vi "DOE Parse Temperature and Voltage.vi"(7 "Test Fixture Hardware":T1={"Power "={"Yokogawa"={"WT210"={"Sample Rate (1: 0.25s)"=1, "A Range (12: 20A)"=11, "V Range (6: 600V)"=4, "Power VISA Yokogawa WT210"="WT210"}, "WT500"={"Power VISA Yokogawa WT500"="", "V Range (8: 1000V)"=6, "I Range (7: 40A)"=7, "Update Rate (3: 500ms)"=2}, "WT310_2"={"Sample Rate (1: 0.25s)"=1, "A Range (12: 20A)"=11, "V Range (6: 600V)"=4, "Power VISA Yokogawa WT310_2"="WT310_2"}, "WT310_3"={"Sample Rate (1: 0.25s)"=1, "A Range (12: 20A)"=11, "V Range (6: 600V)"=4, "Power VISA Yokogawa WT310_3"="WT310_3"}}, "Aplus"={"Aplus IP Address"="192.168.1.101", "Remote Port"=502, "Instrument"="APLUS", "Instr Driver Revision"="1.03.0053"}, "Power Limits"={"Crest Factor"={"Upper Limit"=1.49, "Lower Limit"=1.34}, "Harmonic Content"={"Uthd"=2.0}, "Voltage"={"% Error"=2.0}, "Stability"={"<1 Watt "={"Wattage"=1.0, "Slope (mW/H)"=10.0}, ">1 Watt"={"1%Power/Hour"=1.0}}}, "Nominal Voltage"=120, "Time Limit (s)"=10800.0, "Power Variation Limit (%)"=50.0, "Power Supply"={"Chroma 61605"="CHROMA", "Use Chroma?"=FALSE}}, "Weight Scale"={"Com Options"={"IND560Scale VISA"="IND560", "IP Address"="", "Remote Port"=502, "Setra Scale VISA"="SETRA", "GSE 350"="GSE350"}, "Select Scale"=""}, "Flow Rates"={"Laurel Cold IP Address"="", "Laurel Hot IP Address"="", "Hot Water Laurel VISA"="LaurelMeter_Hot", "Cold Water Laurel VISA"="LaurelMeter_Cold", "Remote Port"=0, "Laurel Communication Type"="", "Meters To Collect (Hot Cold)"="", "HOT Laurel Reference"=refnum, "COLD Laurel Reference"=refnum}, "Analog Data"={"Agilent"={"Agilent 34972_1"="34972A_1", "Agilent 34972_2"="34972A_2", "Agilent 34972_3"="34972A_3", "Agilent 34972_4"="34972A_3", "Agilent 34972_5"="34972A_3", "Agilent 34972_6"="34972A_3", "Agilent Gain"=0.0, "TC Type (K,J,T)"="", "Instrument IDN?"="", "TC Channels-List"="", "Analog Channels-List"="", "Agilent Cluster Array"=[], "TC Channels-List 2"="", "Analog Channels-List 2"=""}, "Yokogawa"={"MW100"="MW100", "Intellifaucet"=FALSE}, "Select Analog"="", "TC Coefficients"={"TC Coefficients 1"=[], "TC Coefficients 2"=[], "TC Coefficients 3"=[], "TC Coefficients 4"=[], "TC Coefficients 5"=[], "TC Coefficients 6"=[], "TC Coefficients 7"=[]}, "NI Tasks (Dryer DOE)"=["TC Temps-Module 1", "TC Temps-Module 2", "TC Temps-Module 3", "TC Temps-Module 4", "TC Temps-Module 5", "Gas and Temp-Module 6", "AC_DC Events-Module 7"], "Laurel Analog"={"Laurel IP (Water Temp)"="", "Laurel IP (Pressure)"=""}}, "ITHX-Temp Humidity"={"IP Address 1"="", "Remote Port"=0, "IP Address 2"="", "IP Address 3"=""}, "Gas Meter COM Ports"={"Gas Meter 1"="COM3", "Gas Meter 2"="COM4", "Gas Meter 3"="COM5", "Gas Meter 4"="COM6", "Gas Meter 5"="COM7", "Gas Meter 6"="COM8"}, "Barometric Pressure"={"HEISE 901A"="HEISE", "Use Barometer?"=FALSE}} {"Power"."Yokogawa"."WT310_3"."V Range (6: 600V)" items=["Auto", "15V", "30V", "60V", "150V", "300V", "600V"]; "Power"."Yokogawa"."WT310_3"."A Range (12: 20A)" items=["Auto", "5mA", "10mA", "20mA", "50mA", "100mA", "200mA", "0.5A", "1A", "2A", "5A", "10A", "20A", "50mV", "100mV", "200mV", "2.5V", "5V", "10V"]; "Power"."Yokogawa"."WT310_3"."Sample Rate (1: 0.25s)" items=["0.1s", "0.25s", "0.5s", "1s", "2s", "5s"]; "Power"."Yokogawa"."WT310_2"."V Range (6: 600V)" items=["Auto", "15V", "30V", "60V", "150V", "300V", "600V"]; "Power"."Yokogawa"."WT310_2"."A Range (12: 20A)" items=["Auto", "5mA", "10mA", "20mA", "50mA", "100mA", "200mA", "0.5A", "1A", "2A", "5A", "10A", "20A", "50mV", "100mV", "200mV", "2.5V", "5V", "10V"]; "Power"."Yokogawa"."WT310_2"."Sample Rate (1: 0.25s)" items=["0.1s", "0.25s", "0.5s", "1s", "2s", "5s"]; "Power"."Yokogawa"."WT500"."Update Rate (3: 500ms)" items=["-", "100ms", "200ms", "500ms", "1s", "2s", "5s"]; "Power"."Yokogawa"."WT500"."I Range (7: 40A)" items=["AUTO", "500 mA", "1 A", "2 A", "5 A", "10 A", "20 A", "40 A", "S-AUTO", "50 mV", "100 mV", "200 mV", "500 mV", "1 V", "2 V", "5 V", "10 V", "250 mA", "500 mA", "1 A", "2.5 A", "5 A", "10 A", "20 A", "25 mV", "50 mV", "100 mV", "250 mV", "500 mV", "1 V", "2.5 V", "5 V"]; "Power"."Yokogawa"."WT500"."V Range (8: 1000V)" items=["AUTO", "15", "30", "60", "100", "150", "300", "600", "1000", "7.5", "15", "30", "50", "75", "150", "300", "500"]; "Power"."Yokogawa"."WT210"."V Range (6: 600V)" items=["Auto", "15V", "30V", "60V", "150V", "300V", "600V"]; "Power"."Yokogawa"."WT210"."A Range (12: 20A)" items=["Auto", "5mA", "10mA", "20mA", "50mA", "100mA", "200mA", "0.5A", "1A", "2A", "5A", "10A", "20A", "50mV", "100mV", "200mV", "2.5V", "5V", "10V"]; "Power"."Yokogawa"."WT210"."Sample Rate (1: 0.25s)" items=["0.1s", "0.25s", "0.5s", "1s", "2s", "5s"]}, 10 "TC Coefficients":T5, 11 "All Data":dbl[](array[numeric])) -> (2 "DOE Agilent Data":string[][](array[string]), 3 "Data Output":T7, 5 "DOE DBL Data":dbl[](array[numeric]))   [LabVIEW 2018]
uses:
  Utility/Type Definitions/UTILITY TC Coefficients.ctl
  Drivers/Advantech/Type Definitions/Advantech DAQ.ctl
  Type Definitions/DOE Test Fixture Hardware.ctl
  Utility/Type Definitions/UTILITY Power Inputs Control.ctl
  Drivers/IND560 Scale Monitor/Type Definitions/IND560 Configuration.ctl
  Hybrid Water Heater/Type Definitions/HEWH Agilent Cluster.ctl
  Drivers/Omega FMA-1600A Series Gas Flow Meter/Type Definitions/FMA1600A COM Ports.ctl
  Utility/Type Definitions/UTILITY TC Coefficients Selector.ctl
panel:
  out "Loop Number":i32
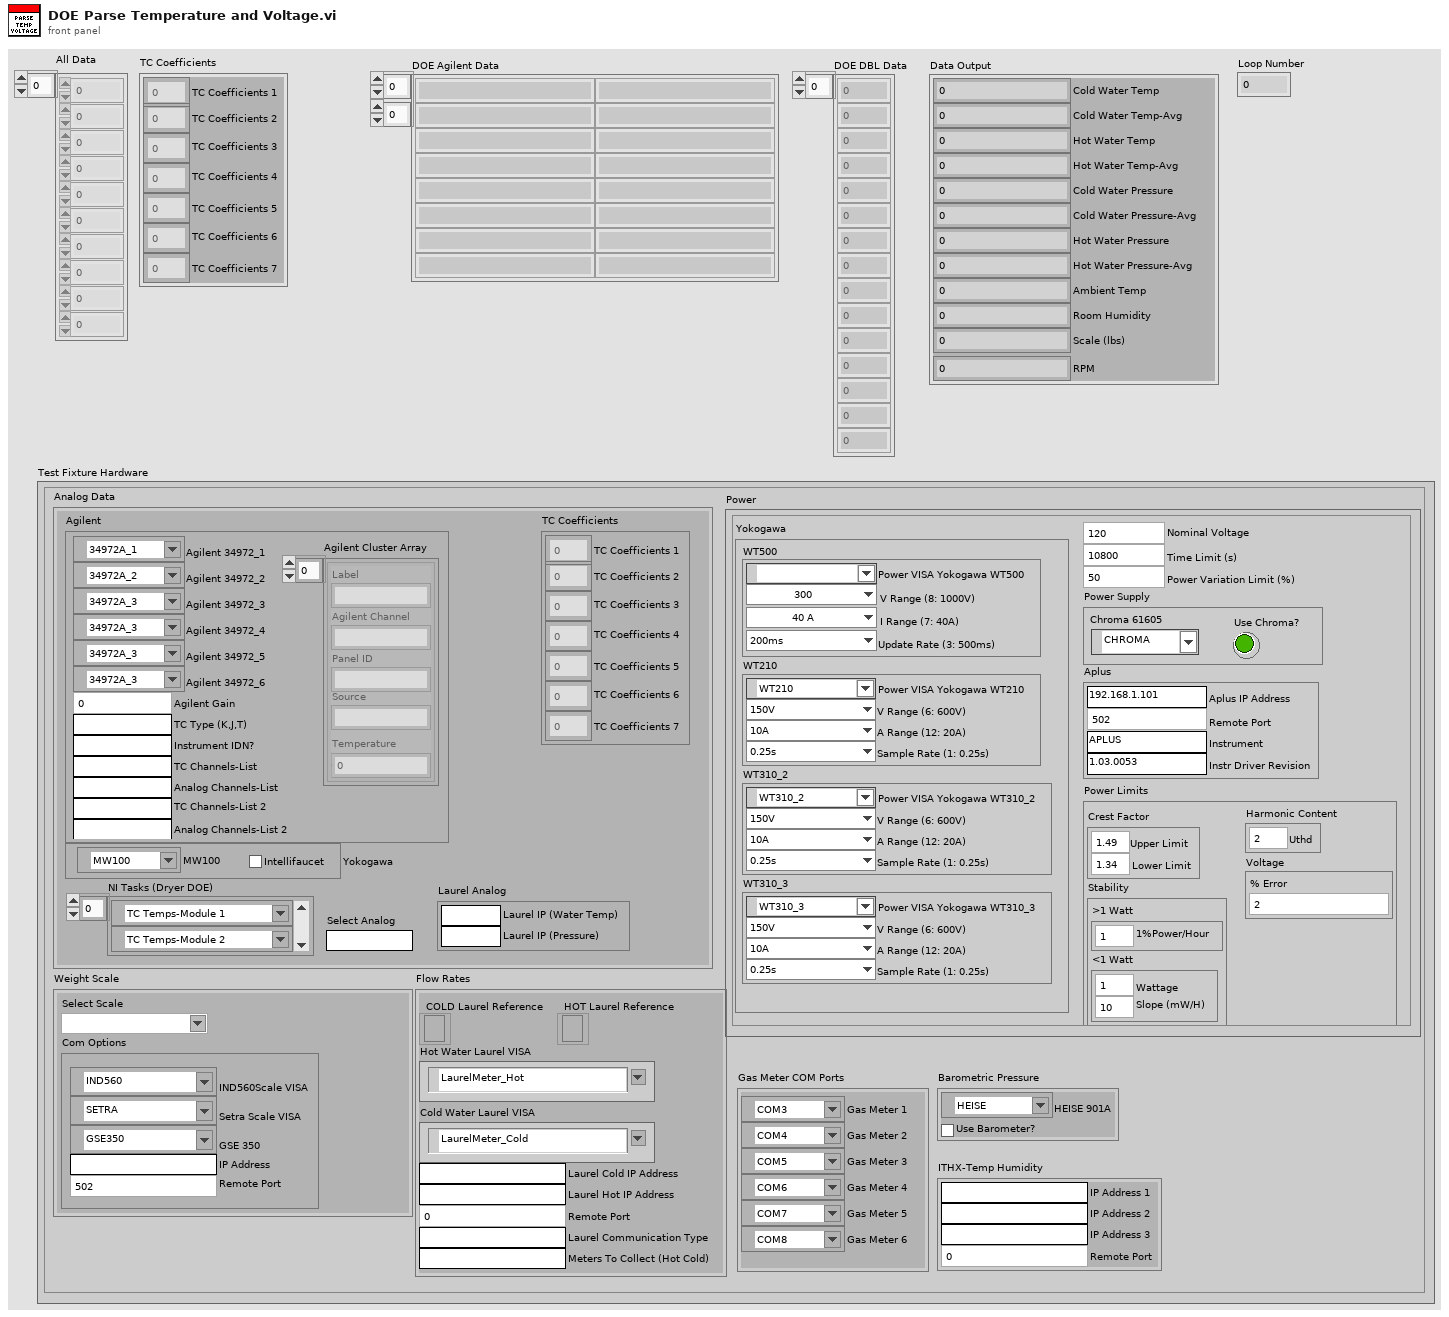
[diagram p1: front panel]
types:
  T1 = typedef "DOE Test Fixture Hardware.ctl" = cluster{"Power ":T2, "Weight Scale":cluster{"Com Options":T3, "Select Scale":string}, "Flow Rates":cluster{"Laurel Cold IP Address":string, "Laurel Hot IP Address":string, "Hot Water Laurel VISA":refnum<visa-resource-name>, "Cold Water Laurel VISA":refnum<visa-resource-name>, "Remote Port":u16, "Laurel Communication Type":string, "Meters To Collect (Hot Cold)":string, "HOT Laurel Reference":refnum<k5>, "COLD Laurel Reference":refnum<k5>}, "Analog Data":cluster{"Agilent":cluster{"Agilent 34972_1":refnum<visa-resource-name>, "Agilent 34972_2":refnum<visa-resource-name>, "Agilent 34972_3":refnum<visa-resource-name>, "Agilent 34972_4":refnum<visa-resource-name>, "Agilent 34972_5":refnum<visa-resource-name>, "Agilent 34972_6":refnum<visa-resource-name>, "Agilent Gain":dbl, "TC Type (K,J,T)":string, "Instrument IDN?":string, "TC Channels-List":string, "Analog Channels-List":string, "Agilent Cluster Array":T4[], "TC Channels-List 2":string, "Analog Channels-List 2":string}, "Yokogawa":cluster{"MW100":refnum<visa-resource-name>, "Intellifaucet":bool}, "Select Analog":string, "TC Coefficients":T5, "NI Tasks (Dryer DOE)":refnum<k21>[], "Laurel Analog":cluster{"Laurel IP (Water Temp)":string, "Laurel IP (Pressure)":string}}, "ITHX-Temp Humidity":cluster{"IP Address 1":string, "Remote Port":u16, "IP Address 2":string, "IP Address 3":string}, "Gas Meter COM Ports":T6, "Barometric Pressure":cluster{"HEISE 901A":refnum<visa-resource-name>, "Use Barometer?":bool}}
  T2 = typedef "UTILITY Power Inputs Control.ctl" = cluster{"Yokogawa":cluster{"WT210":cluster{"Sample Rate (1: 0.25s)":i32, "A Range (12: 20A)":i32, "V Range (6: 600V)":i32, "Power VISA Yokogawa WT210":refnum<visa-resource-name>}, "WT500":cluster{"Power VISA Yokogawa WT500":refnum<visa-resource-name>, "V Range (8: 1000V)":i32, "I Range (7: 40A)":i32, "Update Rate (3: 500ms)":i32}, "WT310_2":cluster{"Sample Rate (1: 0.25s)":i32, "A Range (12: 20A)":i32, "V Range (6: 600V)":i32, "Power VISA Yokogawa WT310_2":refnum<visa-resource-name>}, "WT310_3":cluster{"Sample Rate (1: 0.25s)":i32, "A Range (12: 20A)":i32, "V Range (6: 600V)":i32, "Power VISA Yokogawa WT310_3":refnum<visa-resource-name>}}, "Aplus":cluster{"Aplus IP Address":string, "Remote Port":i32, "Instrument":string, "Instr Driver Revision":string}, "Power Limits":cluster{"Crest Factor":cluster{"Upper Limit":dbl, "Lower Limit":dbl}, "Harmonic Content":cluster{"Uthd":dbl}, "Voltage":cluster{"% Error":dbl}, "Stability":cluster{"<1 Watt ":cluster{"Wattage":dbl, "Slope (mW/H)":dbl}, ">1 Watt":cluster{"1%Power/Hour":dbl}}}, "Nominal Voltage":i32, "Time Limit (s)":dbl, "Power Variation Limit (%)":dbl, "Power Supply":cluster{"Chroma 61605":refnum<visa-resource-name>, "Use Chroma?":bool}}
  T3 = typedef "IND560 Configuration.ctl" = cluster{"IND560Scale VISA":refnum<visa-resource-name>, "IP Address":string, "Remote Port":u16, "Setra Scale VISA":refnum<visa-resource-name>, "GSE 350":refnum<visa-resource-name>}
  T4 = typedef "HEWH Agilent Cluster.ctl" = cluster{"Label":string, "Agilent Channel":string, "Panel ID":string, "Source":string, "Temperature":dbl}
  T5 = typedef "UTILITY TC Coefficients.ctl" = cluster{"TC Coefficients 1":dbl[], "TC Coefficients 2":dbl[], "TC Coefficients 3":dbl[], "TC Coefficients 4":dbl[], "TC Coefficients 5":dbl[], "TC Coefficients 6":dbl[], "TC Coefficients 7":dbl[]}
  T6 = typedef "FMA1600A COM Ports.ctl" = cluster{"Gas Meter 1":refnum<visa-resource-name>, "Gas Meter 2":refnum<visa-resource-name>, "Gas Meter 3":refnum<visa-resource-name>, "Gas Meter 4":refnum<visa-resource-name>, "Gas Meter 5":refnum<visa-resource-name>, "Gas Meter 6":refnum<visa-resource-name>}
  T7 = typedef "Advantech DAQ.ctl" = cluster{"Cold Water Pressure":dbl, "Hot Water Pressure":dbl, "Cold Water Temp":dbl, "Hot Water Temp":dbl, "Ambient Temp":dbl, "Room Humidity":dbl, "Scale (lbs)":dbl, "RPM":dbl, "Cold Water Temp-Avg":dbl, "Hot Water Temp-Avg":dbl, "Cold Water Pressure-Avg":dbl, "Hot Water Pressure-Avg":dbl}
  T8 = typedef "UTILITY TC Coefficients Selector.ctl" = enum16{"TC1", "TC2", "TC3", "TC4", "TC5", "TC6", "TC7"}
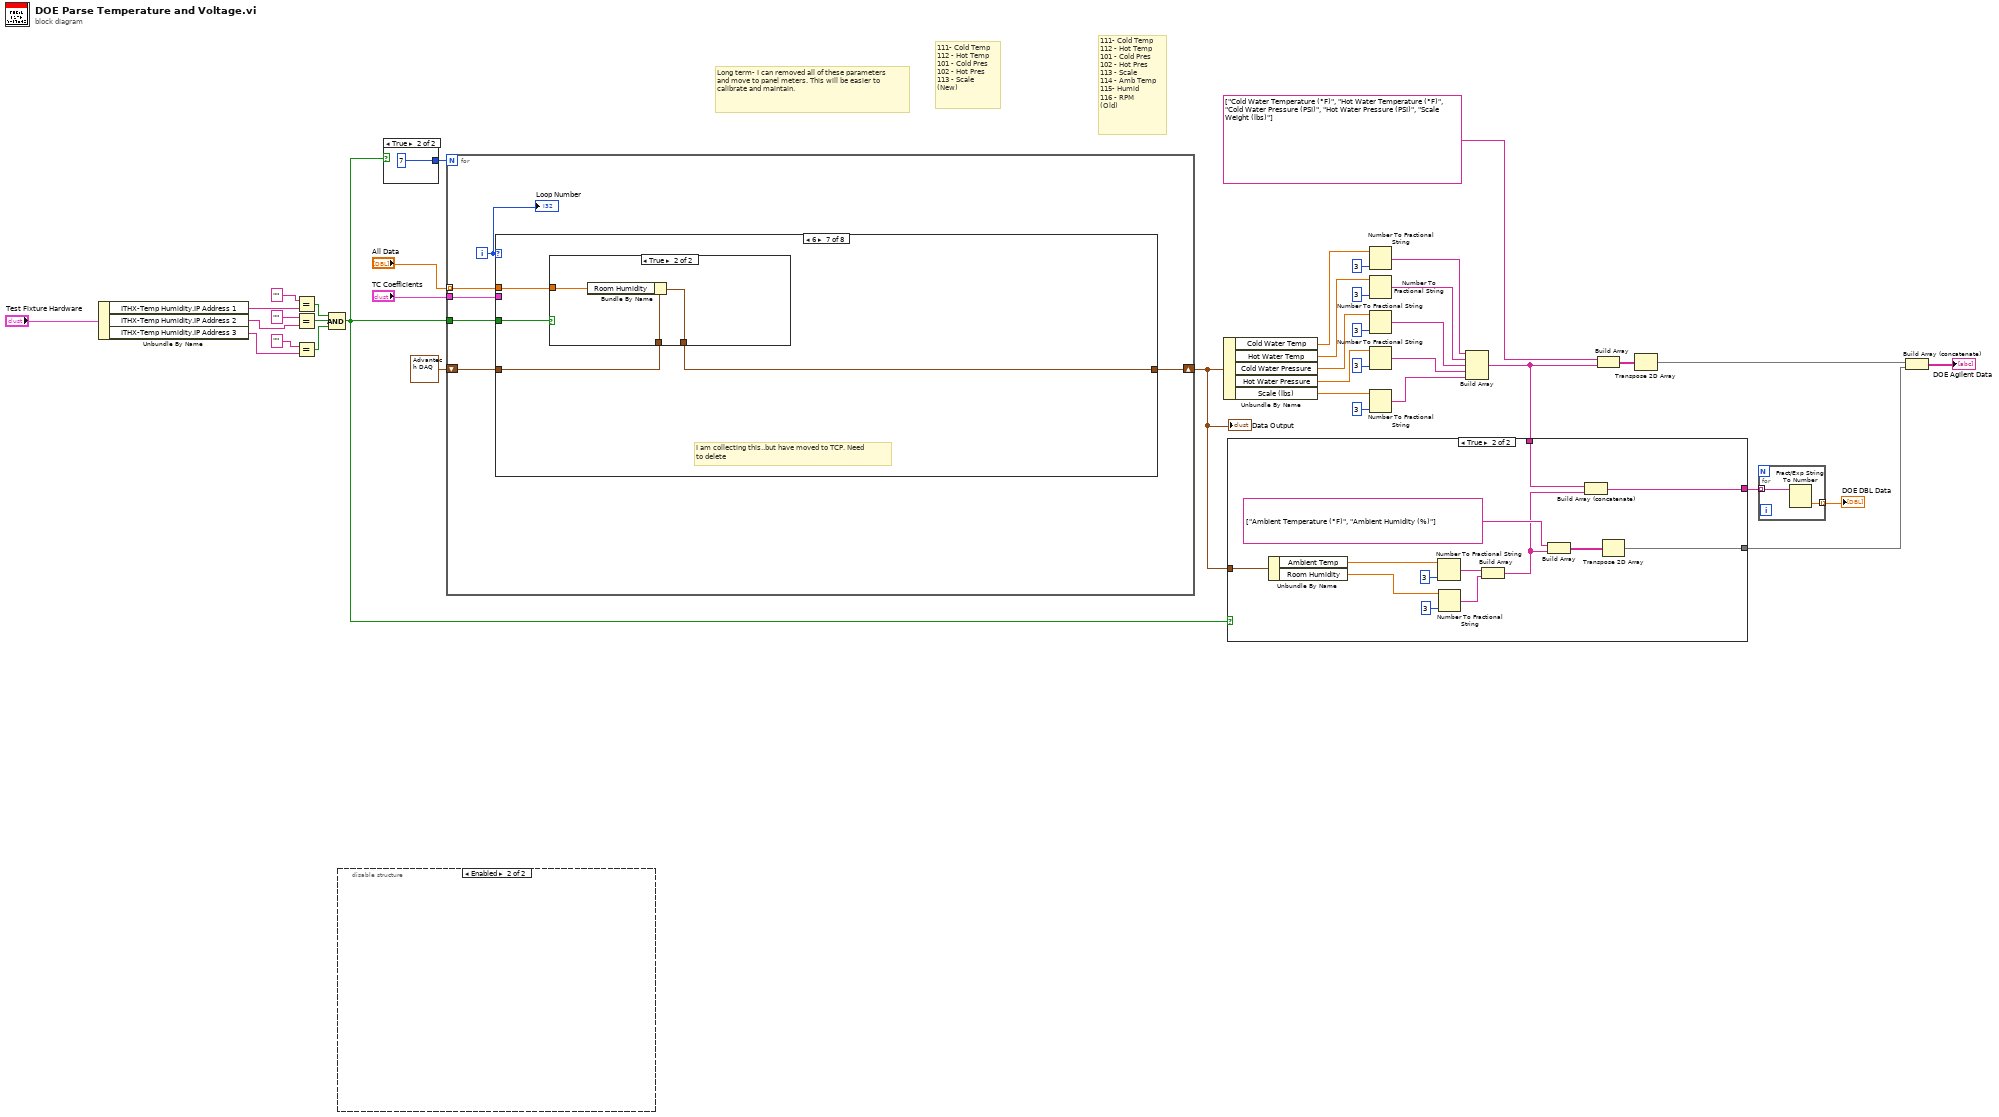
[diagram p0: block diagram]
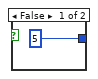
[diagram p2: hidden frame]
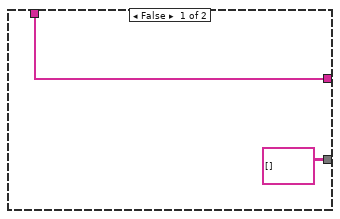
[diagram p3: hidden frame]
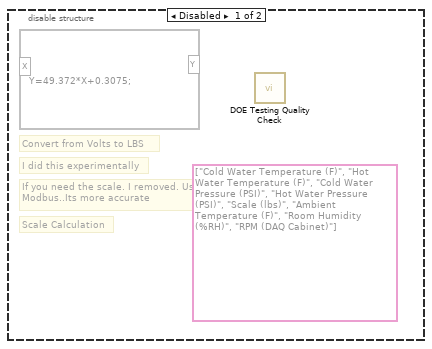
[diagram p4: hidden frame]
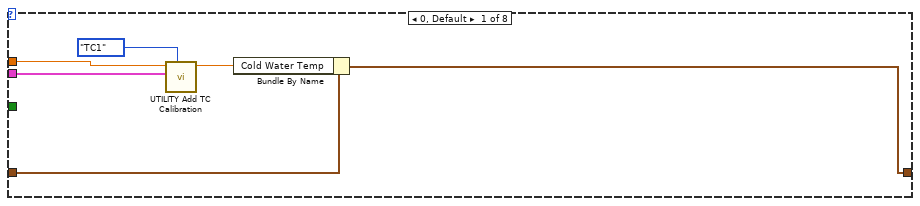
[diagram p5: hidden frame]
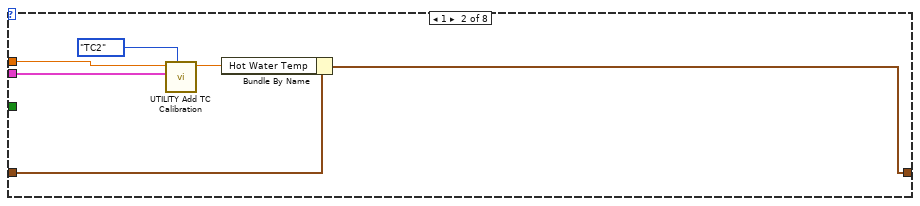
[diagram p6: hidden frame]
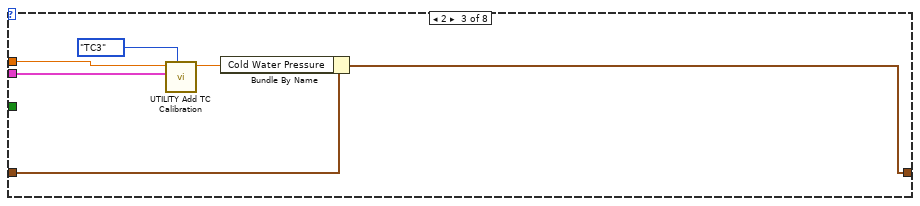
[diagram p7: hidden frame]
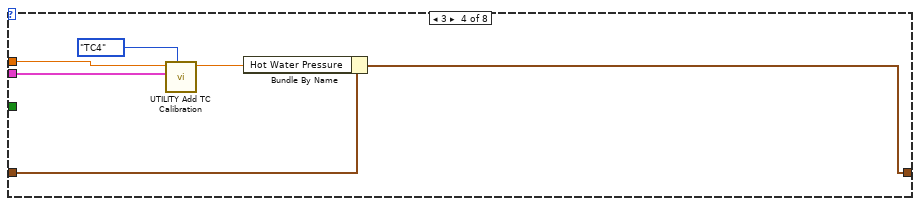
[diagram p8: hidden frame]
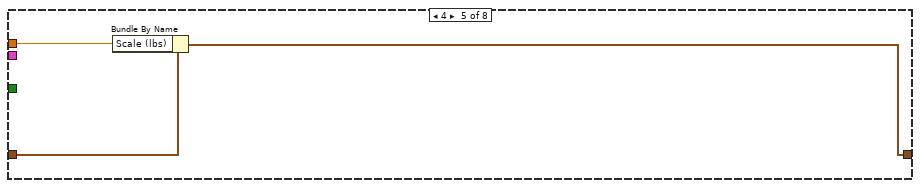
[diagram p9: hidden frame]
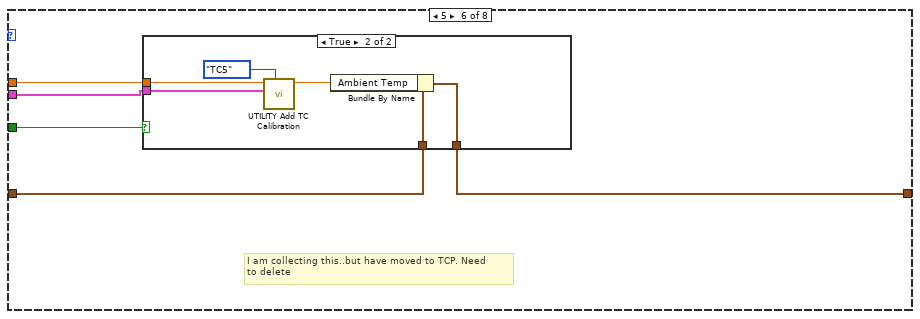
[diagram p10: hidden frame]
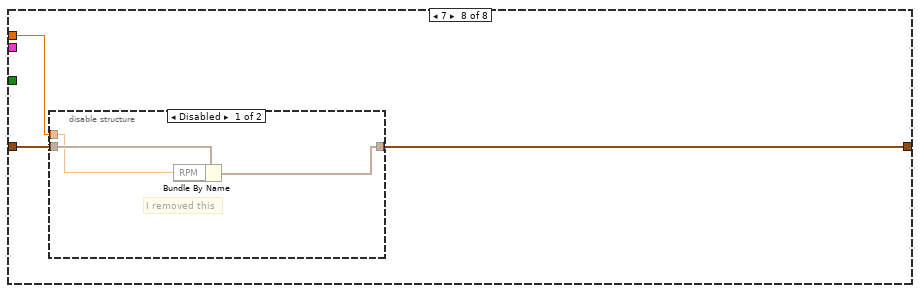
[diagram p13: hidden frame]
diagram:
  # "111- Cold Temp\n112 - Hot Temp\n101 - Cold Pres \n102 - Hot Pres\n113 - Scale\n(New)"
  # "Long term- I can removed all of these parameters\nand move to panel meters. This will be easier to \ncalibrate and maintain."
  # "111- Cold Temp\n112 - Hot Temp\n101 - Cold Pres \n102 - Hot Pres\n113 - Scale\n114 - Amb Temp\n115- Humid\n116 - RPM\n(Old)"
  n1 = Unbundle By Name("Test Fixture Hardware") -> ("ITHX-Temp Humidity.IP Address 1"=w18:string, "ITHX-Temp Humidity.IP Address 2"=w16:string, "ITHX-Temp Humidity.IP Address 3"=w15:string)
  n2 = Equal?(x="" ("y"), y=w18) -> (x = y?=w12:bool)
  n3 = Equal?(x="" ("y"), y=w16) -> (x = y?=w11:bool)
  n4 = Equal?(x="" ("y"), y=w15) -> (x = y?=w10:bool)
  n5 = Compound Arithmetic op=AND(w12, w11, w10) -> (w1:bool)
  n6 = disable-structure shown="Enabled" {
    frame Disabled {
      (unwired) string[] ["Cold Water Temperature (F)", "Hot Water Temperature (F)", "Cold Water Pressure (PSI)", "Hot Water Pressure (PSI)", "Scale (lbs)", "Ambient Temperature (F)", "Room Humidity (%RH)", "RPM (DAQ Cabinet)"]
      # "If you need the scale. I removed. Use\nModbus..Its more accurate"
      # "Convert from Volts to LBS"
      # "I did this experimentally"
      # "Scale Calculation"
      n7 = formula code="Y=49.372*X+0.3075;"() -> ()  [unwired: 1 in, 1 out]
      n8 = call "DOE Testing Quality Check.vi"() -> ()  [unwired: 15 in, 5 out]
    }
    frame Enabled {
    }
  }
  n9 = case shown="True" w1 {
    tunnel: [5 7] -> w2
    frame False {
    }
    frame True {
    }
  }
  n10 = for {
    N: w2 -> [_]
    tunnel: "All Data" -> [w46] mode=indexing
    tunnel: "TC Coefficients" -> [w45]
    shift-right: [w43] -> w9
    shift-left: T7 {"Cold Water Pressure"=0.0, "Hot Water Pressure"=0.0, "Cold Water Temp"=0.0, "Hot Water Temp"=0.0, "Ambient Temp"=0.0, "Room Humidity"=0.0, "Scale (lbs)"=0.0, "RPM"=0.0, "Cold Water Temp-Avg"=0.0, "Hot Water Temp-Avg"=0.0, "Cold Water Pressure-Avg"=0.0, "Hot Water Pressure-Avg"=0.0} ("Advantech") -> [w44]
    tunnel: w1 -> [w42]
    i -> [w47]
    n11 = case shown="6" w47 {
      tunnel: w46 -> [w52 w58 w63 w69 w72 w78 w88 w95]
      tunnel: w45 -> [w53 w57 w64 w70 _ w79 _ _]
      tunnel: w44 -> [w50 w56 w62 w68 w74 w77 w90 w97]
      tunnel: [w49 w55 w61 w67 w73 w76 w89 w96] -> w43
      tunnel: w42 -> [_ _ _ _ _ w75 w87 _]
      frame 0, Default {
        n12 = call "UTILITY Add TC Calibration.vi"("Enum"=UTILITY_TC_Coefficients_Selector."TC1", "TC Coefficients"=w53, "Non Cal Temp"=w52) -> ("Calibrated Temp"=w48:dbl)  [unwired: 8 in]
        n13 = Bundle By Name(cluster=w50, "Cold Water Temp"=w48) -> (w49:T7)
      }
      frame 1 {
        n14 = call "UTILITY Add TC Calibration.vi"("Enum"=UTILITY_TC_Coefficients_Selector."TC2", "TC Coefficients"=w57, "Non Cal Temp"=w58) -> ("Calibrated Temp"=w54:dbl)  [unwired: 8 in]
        n15 = Bundle By Name(cluster=w56, "Hot Water Temp"=w54) -> (w55:T7)
      }
      frame 2 {
        n16 = call "UTILITY Add TC Calibration.vi"("Enum"=UTILITY_TC_Coefficients_Selector."TC3", "TC Coefficients"=w64, "Non Cal Temp"=w63) -> ("Calibrated Temp"=w60:dbl)  [unwired: 8 in]
        n17 = Bundle By Name(cluster=w62, "Cold Water Pressure"=w60) -> (w61:T7)
      }
      frame 3 {
        n18 = call "UTILITY Add TC Calibration.vi"("Enum"=UTILITY_TC_Coefficients_Selector."TC4", "TC Coefficients"=w70, "Non Cal Temp"=w69) -> ("Calibrated Temp"=w66:dbl)  [unwired: 8 in]
        n19 = Bundle By Name(cluster=w68, "Hot Water Pressure"=w66) -> (w67:T7)
      }
      frame 4 {
        n20 = Bundle By Name(cluster=w74, "Scale (lbs)"=w72) -> (w73:T7)
      }
      frame 5 {
        # "I am collecting this..but have moved to TCP. Need\nto delete"
        n21 = case shown="True" w75 {
          tunnel: w79 -> [_ w86]
          tunnel: w78 -> [_ w85]
          tunnel: w77 -> [w80 w84]
          tunnel: [w80 w83] -> w76
          frame False {
          }
          frame True {
            n22 = call "UTILITY Add TC Calibration.vi"("Enum"=UTILITY_TC_Coefficients_Selector."TC5", "TC Coefficients"=w86, "Non Cal Temp"=w85) -> ("Calibrated Temp"=w81:dbl)  [unwired: 8 in]
            n23 = Bundle By Name(cluster=w84, "Ambient Temp"=w81) -> (w83:T7)
          }
        }
      }
      frame 6 {
        # "I am collecting this..but have moved to TCP. Need\nto delete"
        n24 = case shown="True" w87 {
          tunnel: w90 -> [w91 w94]
          tunnel: [w91 w93] -> w89
          tunnel: w88 -> [_ w92]
          frame False {
          }
          frame True {
            n25 = Bundle By Name(cluster=w94, "Room Humidity"=w92) -> (w93:T7)
          }
        }
      }
      frame 7 {
        n26 = disable-structure shown="Disabled" {
          disable-tunnel: w97 -> [w100 w101]
          disable-tunnel: [w99 w101] -> w96
          disable-tunnel: w95 -> [w98 _]
          frame Disabled {
            # "I removed this"
            n27 = Bundle By Name(cluster=w100, "RPM"=w98) -> (w99:T7)
          }
          frame Enabled {
          }
        }
      }
    }
    "Loop Number" <- w47
  }
  "Data Output" <- w9
  n28 = Unbundle By Name(w9) -> ("Cold Water Temp"=w24:dbl, "Hot Water Temp"=w21:dbl, "Cold Water Pressure"=w23:dbl, "Hot Water Pressure"=w22:dbl, "Scale (lbs)"=w25:dbl)
  n29 = Number To Fractional String(number=w24, precision (6)=i16 3) -> (F-format string=w38:string)  [unwired: 2 in]
  n30 = Number To Fractional String(number=w21, precision (6)=i16 3) -> (F-format string=w37:string)  [unwired: 2 in]
  n31 = Number To Fractional String(number=w23, precision (6)=i16 3) -> (F-format string=w36:string)  [unwired: 2 in]
  n32 = Number To Fractional String(number=w22, precision (6)=i16 3) -> (F-format string=w35:string)  [unwired: 2 in]
  n33 = Number To Fractional String(number=w25, precision (6)=i16 3) -> (F-format string=w26:string)  [unwired: 2 in]
  n34 = Build Array(w38, w37, w36, w35, w26) -> (w8:string[])
  n35 = case shown="True" w1 {
    tunnel: w9 -> [_ w108]
    tunnel: w8 -> [w103 w106]
    tunnel: [w103 w105] -> w6
    tunnel: [string[][] [] w104] -> w4
    frame False {
    }
    frame True {
      n36 = Unbundle By Name(w108) -> ("Ambient Temp"=w114:dbl, "Room Humidity"=w113:dbl)
      n37 = Number To Fractional String(number=w114, precision (6)=i16 3) -> (F-format string=w112:string)  [unwired: 2 in]
      n38 = Number To Fractional String(number=w113, precision (6)=i16 3) -> (F-format string=w111:string)  [unwired: 2 in]
      n39 = Build Array(w112, w111) -> (w107:string[])
      n40 = Build Array(string[] ["Ambient Temperature (°F)", "Ambient Humidity (%)"], w107) -> (w109:string[][])
      n41 = Build Array (concatenate)(w106, w107) -> (w105:string[])
      n42 = Transpose 2D Array(2D array=w109) -> (transposed array=w104:string[][])
    }
  }
  n43 = Build Array(string[] ["Cold Water Temperature (°F)", "Hot Water Temperature (°F)", "Cold Water Pressure (PSI)", "Hot Water Pressure (PSI)", "Scale Weight (lbs)"], w8) -> (w33:string[][])
  n44 = Transpose 2D Array(2D array=w33) -> (transposed array=w5:string[][])
  n45 = for {
    tunnel: w6 -> [w118] mode=indexing
    tunnel: [w117] -> w7 mode=indexing
    n46 = Fract/Exp String To Number(string=w118) -> (number=w117:dbl)  [unwired: 3 in, 1 out]
  }
  "DOE DBL Data" <- w7
  n47 = Build Array (concatenate)(w5, w4) -> (→"DOE Agilent Data":string[][])
